vi "Grabber Control.vi"(1 "Forcing":bool, 2 "Holding Button":bool) -> ()   [LabVIEW 2013]
uses:
  <vilib>/Rock Robotics/WPI/Solenoid/WPI_SolenoidValue.ctl
  Robot Global Data.vi
  <vilib>/Rock Robotics/WPI/Solenoid/WPI_SolenoidSetEnum.vi
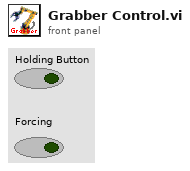
[diagram p1: front panel]
types:
  T1 = typedef "WPI_SolenoidValue.ctl" = enum16{"Off", "On", "Forward", "Reverse"}
  T2 = typedef "WPI_DigitalInputDevRef.ctl" = cluster{"DevStatus":errorcluster, "DIO Channel":T3, "Digital Module":T4}
  T3 = typedef "FPGA_DIOChannel.ctl" = enum8{"DIO 1", "DIO 2", "DIO 3", "DIO 4", "DIO 5", "DIO 6", "DIO 7", "DIO 8", "DIO 9", "DIO 10", "DIO 11", "DIO 12", "DIO 13", "DIO 14", "Invalid"}
  T4 = typedef "FPGA_TypedefDigitalModule.ctl" = enum16{"Digital Module 1", "Digital Module 2"}
  T5 = typedef "WPI_SolenoidDevRef.ctl" = cluster{"DevStatus":errorcluster, "Solenoid Module":T6, "Forward Solenoid Channel":T7, "Reverse Solenoid Channel":T7}
  T6 = typedef "FPGA_TypedefSolenoidModule.ctl" = enum16{"Solenoid Module 1", "Solenoid Module 2"}
  T7 = typedef "WPI_SolenoidChannel.ctl" = enum8{"Solenoid 1", "Solenoid 2", "Solenoid 3", "Solenoid 4", "Solenoid 5", "Solenoid 6", "Solenoid 7", "Solenoid 8", "Invalid"}
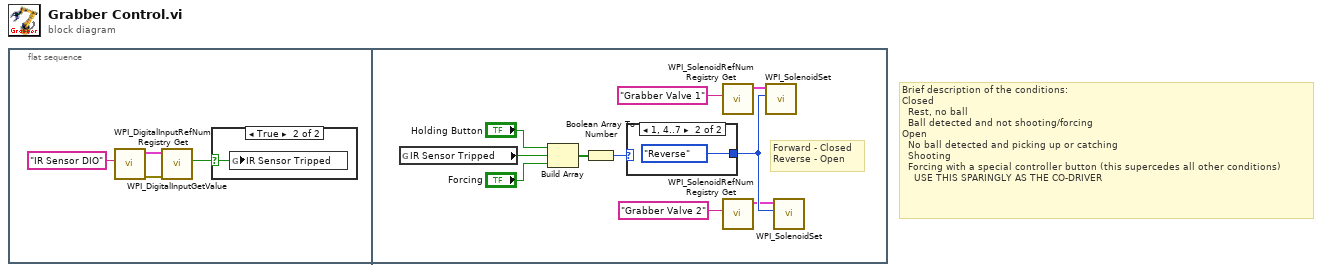
[diagram p0: block diagram]
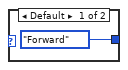
[diagram p3: hidden frame]
diagram:
  # "Brief description of the conditions:\nClosed\n  Rest, no ball\n  Ball detected and not shooting/forcing\nOpen\n  No ball detected and picking up or catching\n  Shooting\n  Forcing with a special controller button (this supercedes all other conditions)\n    USE THIS SPARINGLY AS THE CO-DRIVER"
  n1 = flat-sequence {
    frame #0 {
      n2 = call <vilib>:"WPI_DigitalInputRefNum Registry Get.vi"("refnum name"="IR Sensor DIO") -> ("error out"=w2:errorcluster, "DigitalInputDevRef"=w3:T2)  [unwired: 9 in]
      n3 = call <vilib>:"WPI_DigitalInputGetValue.vi"("error in (no error)"=w2, "DigitalInputDevRef"=w3) -> ("Value"=w4:bool)  [unwired: 7 in, 2 out]
      n4 = case shown="True" w4 {
        selector: w4 -> [_ w5]
        frame False {
        }
        frame True {
          n5 = global write "Robot Global Data.vi" "IR Sensor Tripped"(w5) -> ()
        }
      }
    }
    frame #1 {
      # "Forward - Closed\nReverse - Open"
      n6 = global read "Robot Global Data.vi" "IR Sensor Tripped"() -> (w15:bool)
      n7 = Build Array("Holding Button", w15, "Forcing") -> (w12:bool[])
      n8 = Boolean Array To Number(Boolean array=w12) -> (number=w13:u32)
      n9 = case shown="1, 4..7" w13 {
        tunnel: [WPI_SolenoidValue."Forward" ("Value") WPI_SolenoidValue."Reverse" ("Value")] -> w14
        frame Default {
        }
        frame 1, 4..7 {
        }
      }
      n10 = call <vilib>:"WPI_SolenoidRefNum Registry Get.vi"("refnum name"="Grabber Valve 1") -> ("SolenoidDevRef"=w9:T5)  [unwired: 9 in, 1 out]
      n11 = call <vilib>:"WPI_SolenoidRefNum Registry Get.vi"("refnum name"="Grabber Valve 2") -> ("SolenoidDevRef"=w8:T5)  [unwired: 9 in, 1 out]
      n12 = call-poly <vilib>:"WPI_SolenoidSet.vi"("Value"=w14, "SolenoidDevRef"=w9) -> ()  [unwired: 8 in, 2 out]
      n13 = call-poly <vilib>:"WPI_SolenoidSet.vi"("Value"=w14, "SolenoidDevRef"=w8) -> ()  [unwired: 8 in, 2 out]
    }
  }
